vi "Configure Basic Network Connection.vi"(4 "DHCP (Enabled)":bool=TRUE, 5 "NameServer2 (0.0.0.0)":string="0.0.0.0", 6 "Net Mask (255.255.255.0)":string="255.255.255.0", 7 "NameServer1 (192.168.0.1)":string="192.168.0.1", 8 "error in (no error)":errorcluster, 9 "Gateway Address (192.168.0.1)":string="192.168.0.1", 10 "IP Address (192.168.0.112)":string="192.168.0.112", 11 "VISA resource name":refnum<visa-resource-name>) -> (0 "error out":errorcluster, 3 "VISA resource name out":refnum<visa-resource-name>)   [LabVIEW 2013, in "Watts Up PRO Net Series.lvlib"]
doc: "Basic network configuration for the Watts Up .Net device. Enter your network information in the controls.\n\n<b>Note:</b> The Watts Up .Net will by default find and set these parameters to the device when you connect it to an ethernet port. But if you need to configure them manually then use this VI."
uses:
  <instrlib>/Watts Up PRO Net Series/Watts Up PRO Net Series.lvlib
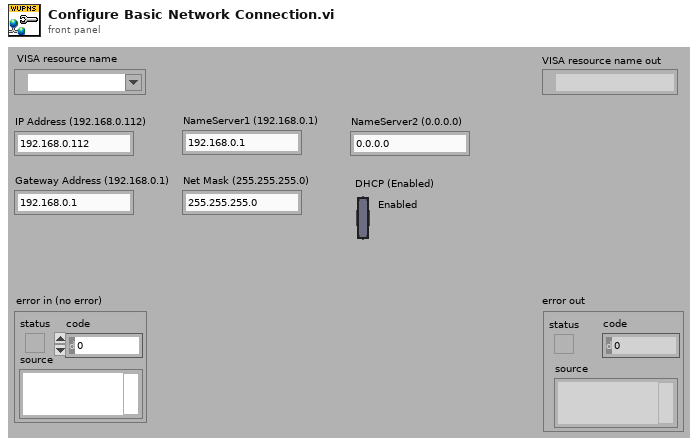
[diagram p1: front panel]
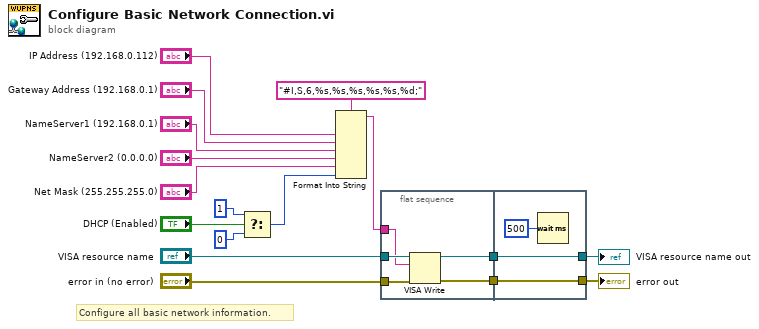
[diagram p0: block diagram]
diagram:
  # "Configure all basic network information."
  n1 = Select(t=1, s="DHCP (Enabled)", f=0) -> (s? t:f=w8:i32)
  n2 = Format Into String(format string="#I,S,6,%s,%s,%s,%s,%s,%d;", "IP Address (192.168.0.112)", "Gateway Address (192.168.0.1)", "NameServer1 (192.168.0.1)", "NameServer2 (0.0.0.0)", "Net Mask (255.255.255.0)", w8) -> (resulting string=w1:string)  [unwired: 2 in, 1 out]
  n3 = flat-sequence {
    tunnel: "VISA resource name" -> [w22]
    tunnel: "error in (no error)" -> [w21]
    tunnel: [w20] -> w3
    tunnel: [w19] -> w2
    tunnel: w1 -> [w18]
    tunnel: [w24] -> w4
    tunnel: [w25] -> w5
    tunnel: w3 -> [w25]
    tunnel: w2 -> [w24]
    frame #0 {
      n4 = VISA Write(VISA resource name=w22, write buffer=w18, error in (no error)=w21) -> (VISA resource name out=w20:refnum<visa-resource-name>, error out=w19:errorcluster)  [unwired: 1 out]
    }
    frame #1 {
      n5 = Wait (ms)(milliseconds to wait=u32 500) -> ()  [unwired: 1 out]
    }
  }
  "VISA resource name out" <- w5
  "error out" <- w4
